vi "LTS60_Set_Current.vi"(8 "error in (no error)":errorcluster, 10 "Beam":bool, 11 "VISA IN":refnum<visa-resource-name>) -> (0 "error out":errorcluster, 3 "VISA resource name out":refnum<visa-resource-name>)   [LabVIEW 2019]
panel:
  out "read buffer":string
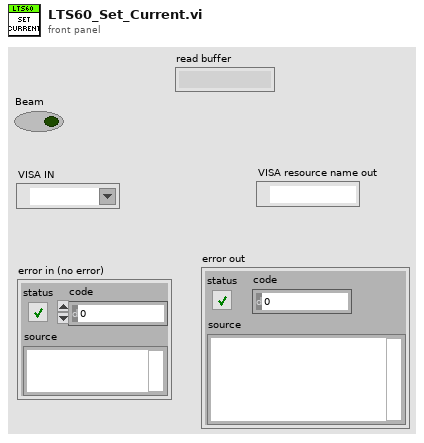
[diagram p1: front panel]
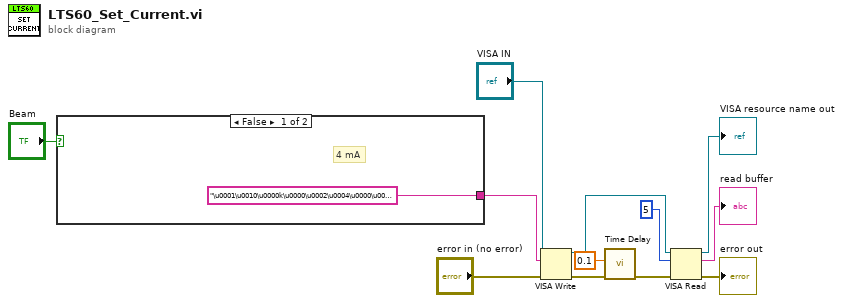
[diagram p0: block diagram]
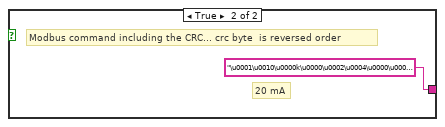
[diagram p2: hidden frame]
diagram:
  n1 = case shown="False" "Beam" {
    tunnel: ["\u0001\u0010\u0000k\u0000\u0002\u0004\u0000\u0000\u0000\u0000´4" ("write buffer") "\u0001\u0010\u0000k\u0000\u0002\u0004\u0000\u0000\u0004胺@" ("write buffer")] -> w11
    frame False {
      # "4 mA"
    }
    frame True {
      # "Modbus command including the CRC... crc byte  is reversed order"
      # "20 mA"
    }
  }
  n2 = VISA Write(VISA resource name="VISA IN", write buffer=w11, error in (no error)="error in (no error)") -> (VISA resource name out=w8:refnum<visa-resource-name>, error out=w10:errorcluster)  [unwired: 1 out]
  n3 = call "Time Delay"("error in (no error)"=w10, "Delay Time (s)"=0.1) -> ("error out"=w9:errorcluster)  [unwired: 9 in]
  n4 = VISA Read(VISA resource name=w8, byte count=u32 5, error in (no error)=w9) -> (VISA resource name out=→"VISA resource name out":refnum<visa-resource-name>, read buffer=→"read buffer":string, error out=→"error out":errorcluster)  [unwired: 1 out]
